vi "Change CH to CH Name.vi"(8 "error in (no error)":errorcluster, 9 "Old #":i32, 10 "New #":i32, 11 "Node Ptr":T1 format="%.0x") -> (0 "error out":errorcluster, 3 "Node Ptr out":T1 format="%.0x")   [LabVIEW 2011, in "NI 272x Resistive Simulation Custom Device Configuration.lvlib"]
uses:
  NI 272x Resistive Simulation Custom Device Configuration.lvlib
  <vilib>/NI Veristand/Custom Device API/Custom Device Item Ref.ctl
  <vilib>/NI Veristand/Custom Device API/Custom Device API.lvlib
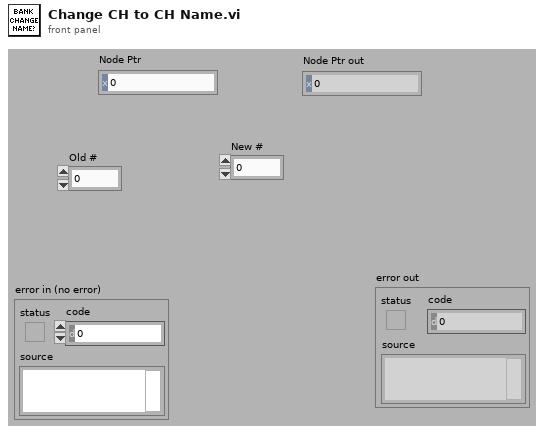
[diagram p1: front panel]
types:
  T1 = typedef "Custom Device API.lvlib/Custom Device Item Ref.ctl" = u64
  T2 = typedef "Custom Device API.lvlib/Custom Device Item Info.ctl" = cluster{"Name":string, "Is Channel":bool, "GUID":string}
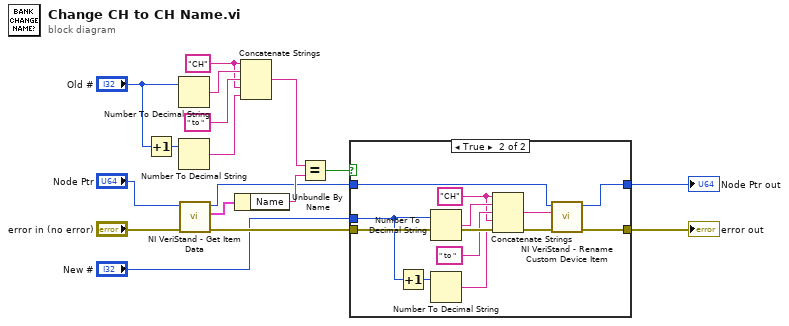
[diagram p0: block diagram]
diagram:
  w4 = "CH"
  n1 = Increment(x="Old #") -> (x+1=w6:i32)
  n2 = Number To Decimal String(number="Old #") -> (decimal integer string=w7:string)  [unwired: 1 in]
  n3 = Number To Decimal String(number=w6) -> (decimal integer string=w3:string)  [unwired: 1 in]
  n4 = call <vilib>:"NI VeriStand - Get Item Data.vi"("error in (no error)"="error in (no error)", "Item Ref in"="Node Ptr") -> ("error out"=w13:errorcluster, "Item Info"=w16:T2, "Item Ref out"=w12:T1)  [unwired: 7 out]
  n5 = Unbundle By Name(w16) -> ("Name"=w14:string)
  n6 = Concatenate Strings(w4, w7, " to ", w4, w3) -> (w1:string)
  n7 = Equal?(x=w1, y=w14) -> (x = y?=w9:bool)
  n8 = case shown="True" w9 {
    tunnel: w13 -> [w19 w30]
    tunnel: w12 -> [w18 w29]
    tunnel: [w18 w28] -> w11
    tunnel: [w19 w27] -> w10
    tunnel: "New #" -> [_ w21]
    frame False {
    }
    frame True {
      w23 = "CH"
      n9 = Increment(x=w21) -> (x+1=w25:i32)
      n10 = Number To Decimal String(number=w21) -> (decimal integer string=w26:string)  [unwired: 1 in]
      n11 = Number To Decimal String(number=w25) -> (decimal integer string=w22:string)  [unwired: 1 in]
      n12 = Concatenate Strings(w23, w26, " to ", w23, w22) -> (w20:string)
      n13 = call <vilib>:"NI VeriStand - Rename Custom Device Item.vi"("error in (no error)"=w30, "New Name"=w20, "Item Ref in"=w29) -> ("error out"=w27:errorcluster, "Item Ref out"=w28:T1)  [unwired: 7 out]
    }
  }
  "error out" <- w10
  "Node Ptr out" <- w11
